vi "内置参数设置.vi"() -> ()   [LabVIEW 2016, in "斯坦道CODMn新电路板.lvlib"]
uses:
  <vilib>/Utility/miscctls.llb/LVPointTypeDef.ctl
panel:
  in  "传感器阈值:":u16
  in  "加速模式(速度):":u16
  in  "滴定延时时间:\n(单位:毫秒)":u16
  in  "斜率阈值:":dbl
  in  "阀配置:":u8(ring) items=["三通阀", "排阀"]
  in  "AB跨度告警值:":u16
  in  "B值告警上限值:":u16
  in  "B值范围:":u16
  in  "A值告警上限值:":u16
  in  "A值范围:":u16
  in  "是否存在液位检测板:":u16(ring) items=["否", "是"]
  in  "检出限(mg/L):":dbl
  in  "测量精度(mg/L):":dbl
  in  "ILimitDown":dbl
  in  "ILimitUp:":dbl
  in  "K d:":dbl
  in  "K i:":dbl
  in  "K p:":dbl
  in  "加热超时时间:(单位:秒)":dbl
  in  "告警温度:":dbl
  in  "加热温度:  校准参数":dbl
  in  "运行速度:  (修改需要重启)":u16
  in  "偏心轮: 校准参数":dbl
  in  "注射泵加热超时时间(s):":u16
  in  "注射泵保温温度H:":u8
  in  "注射泵\n保温温度L:":u8
  in  "废液通道:":u8
  in  "纯水通道:":u8
  in  "滴定速度:":u16
  in  "出样速度:":u16
  in  "进样速度:":u16
  in  "阀数量:":u8(ring) items=["9通"=9, "12通"=12]
  in  "注射泵型号":u8(ring) items=["TECAN", "润泽", "旋转阀"]
  in  "阈值(高→低)(mg/L):":dbl
  in  "阈值(低→高)(mg/L):":dbl
  in  "检测下限(mg/L):":dbl
  in  "检测上限(mg/L):":dbl
  in  "关闭":bool
  in  "保存":bool
  in  "读取":bool
  # "仪器内部参数设置"
  # "~"
  # "~"
  # "~"
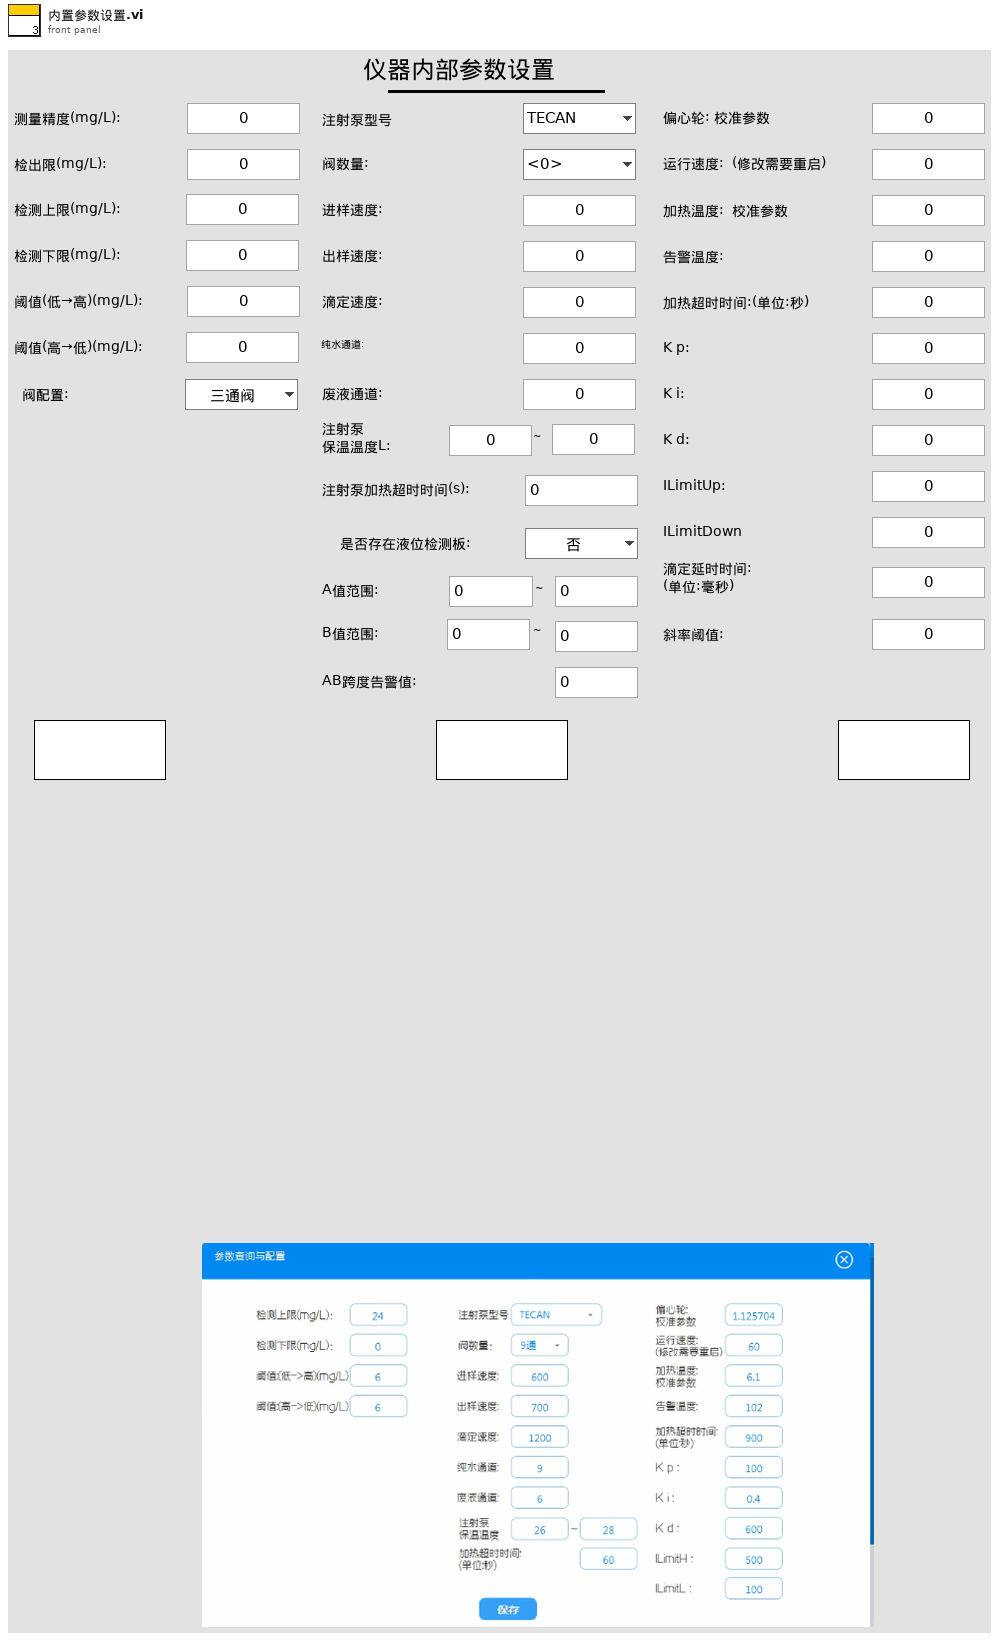
[diagram p1: front panel]
types:
  T1 = typedef "LVPointTypeDef.ctl" = cluster{"Horizontal":i16, "Vertical":i16}
  T2 = cluster{"偏心轮校准参数":dbl, "运行速度(修改需要重启)":u16, "加热温度(校准参数) ":dbl, "告警温度":dbl, "加热超时时间:(单位/秒)":dbl, "K p":dbl, "K i":dbl, "K d":dbl, "ILimitUp":dbl, "ILimitDown":dbl}
  T3 = cluster{"泵类型":u8, "阀数量":u8, "纯水通道":u8, "废液通道":u8, "进样速度":u16, "出样速度":u16, "滴定速度":u16, "注射泵保温温度L":u8, "注射泵保温温度H":u8, "注射泵加热超时时间":u16, "是否存在液位检测板":u16, "A值告警下限值":u16, "A值告警上限值":u16, "B值告警下限值":u16, "B值告警上限值":u16, "AB跨度告警值":u16, "阀配置:":u8, "滴定等待时间":u16, "滴定吸光度斜率":dbl, "传感器阈值":u16, "加速模式(速度):":u16}
  T4 = cluster{"检出限":dbl, "测量精度":dbl, "上限":dbl, "下限":dbl, "阈值（低->高）":dbl, "阈值（高->低）":dbl}
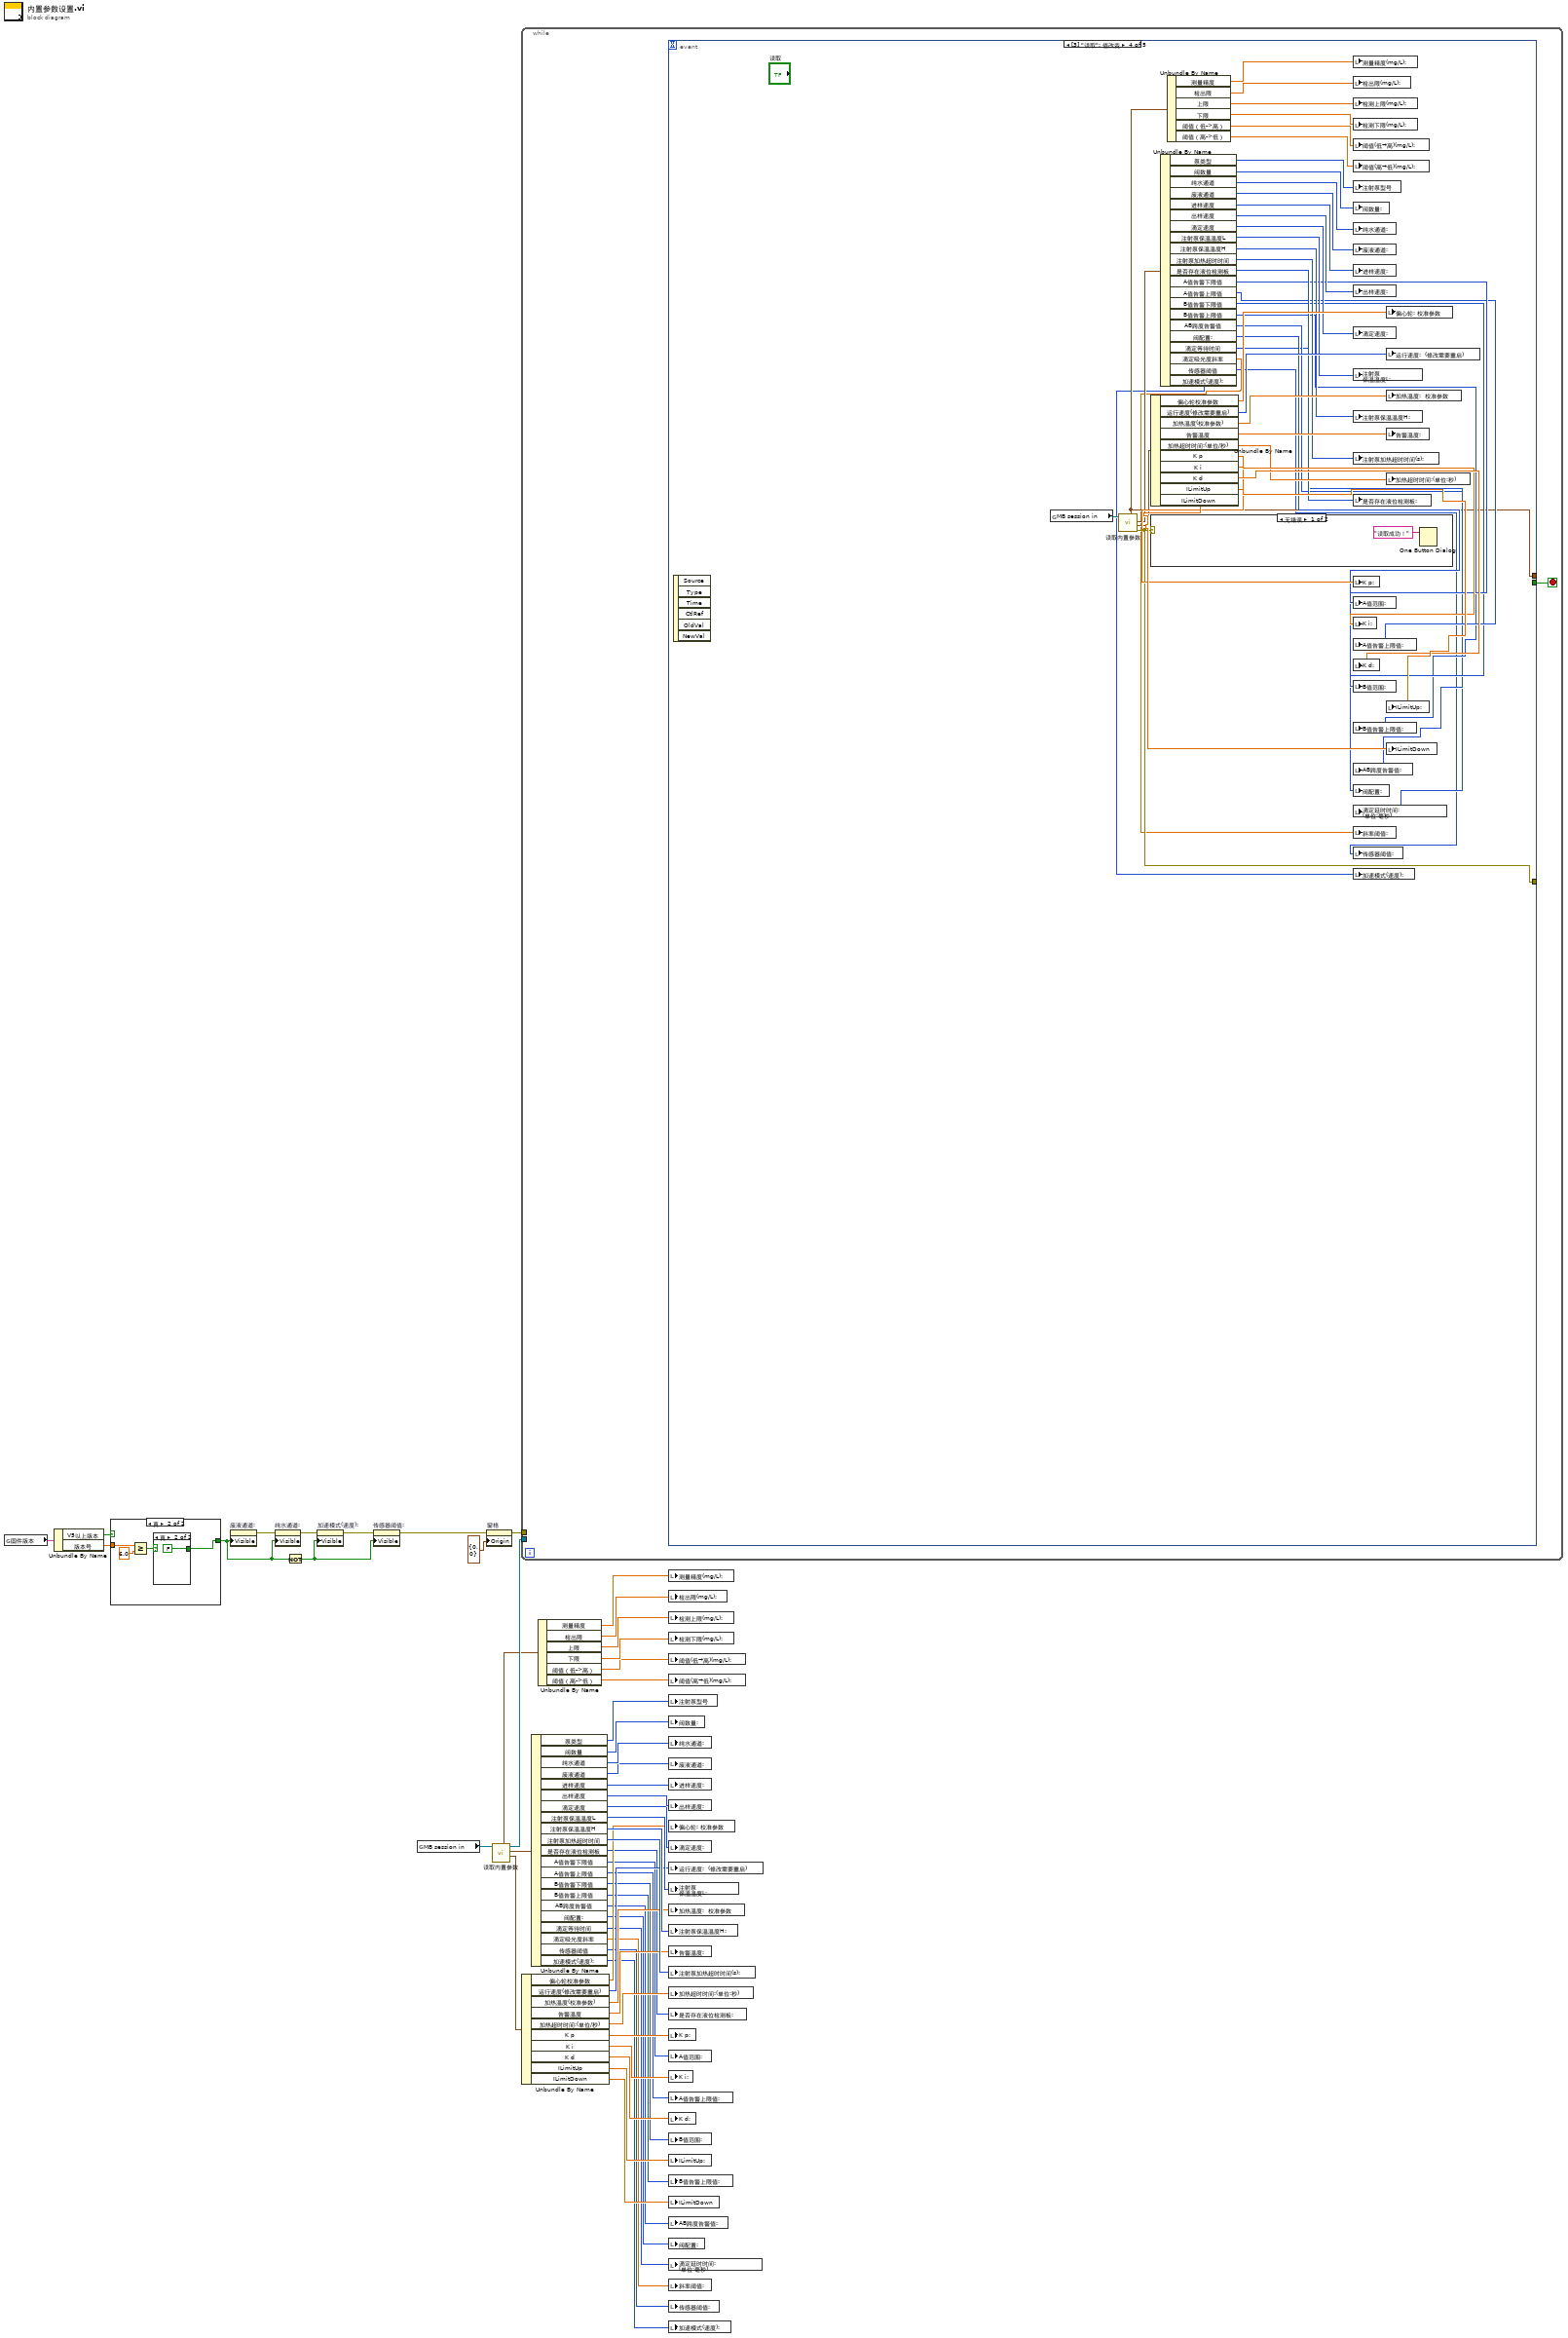
[diagram p0: block diagram]
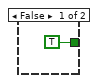
[diagram p2: hidden frame]
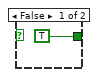
[diagram p3: hidden frame]
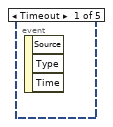
[diagram p4: hidden frame]
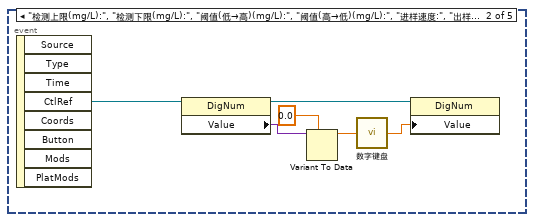
[diagram p5: hidden frame]
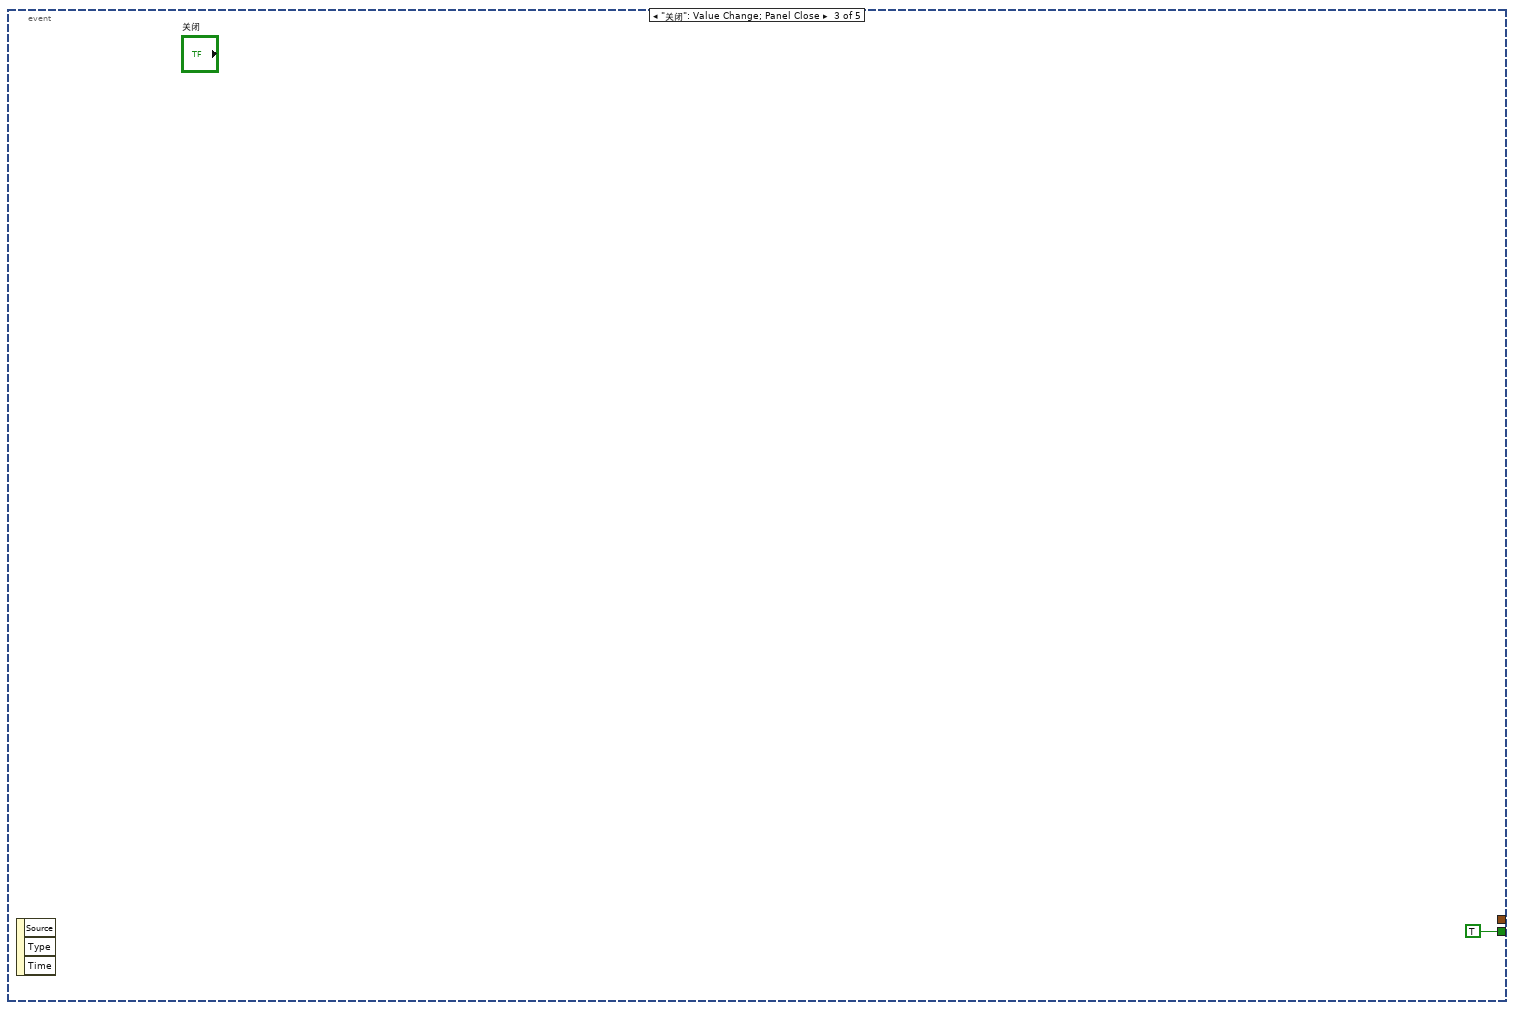
[diagram p6: hidden frame]
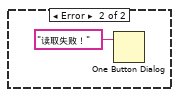
[diagram p7: hidden frame]
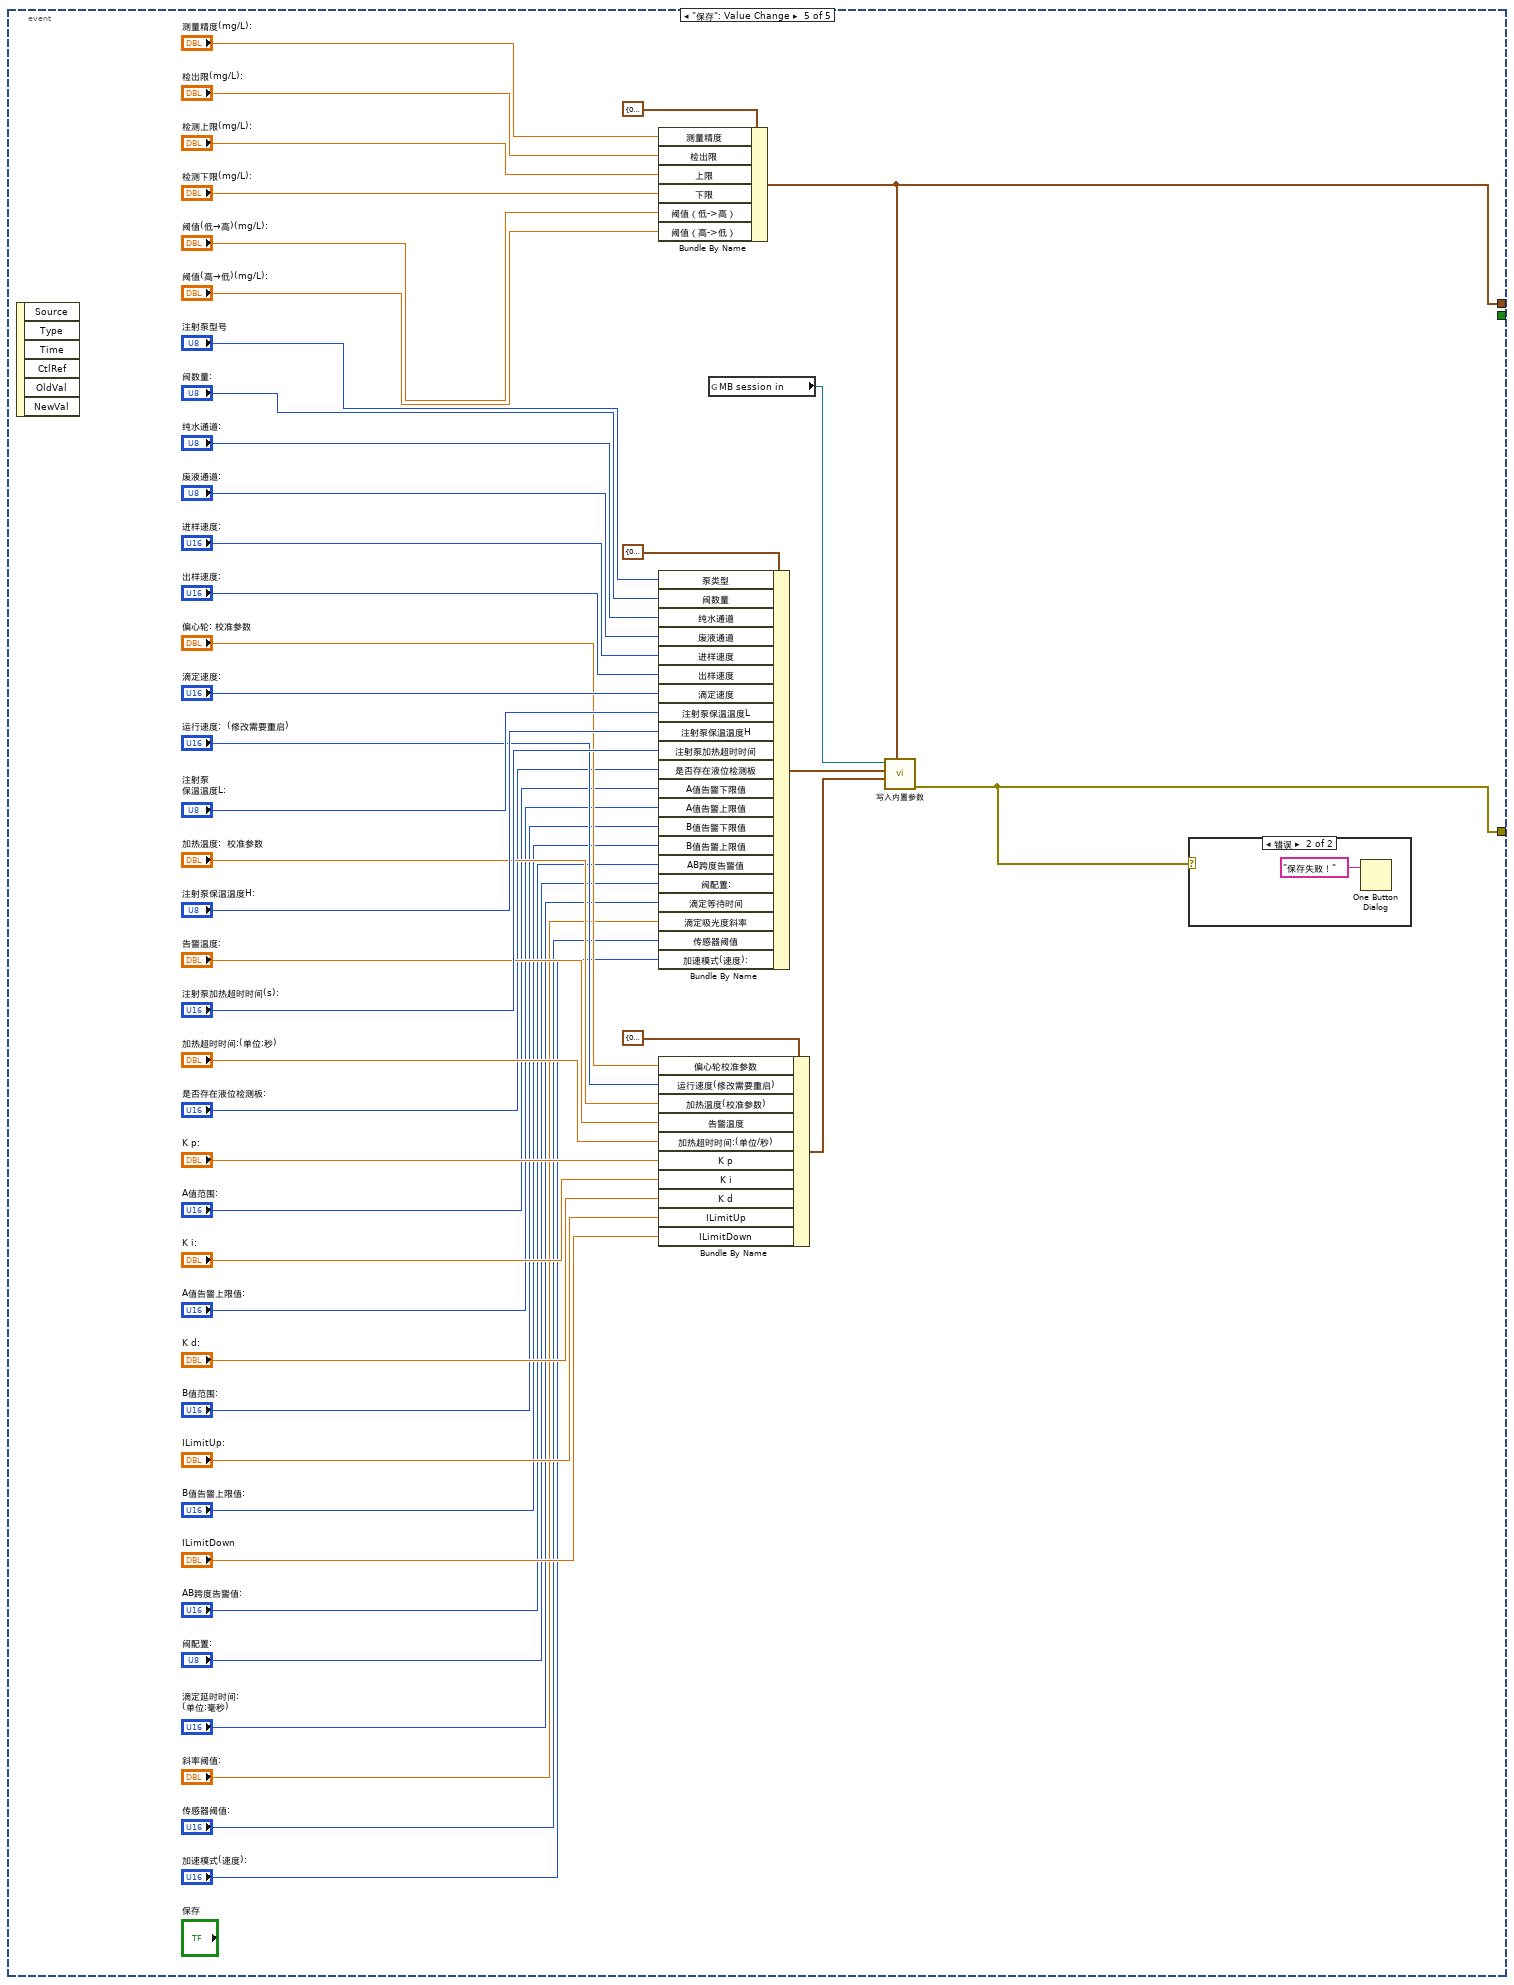
[diagram p8: hidden frame]
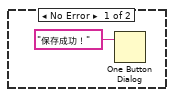
[diagram p9: hidden frame]
diagram:
  n1 = global read "VARCODMn全局变量.vi" "固件版本"() -> (w11:cluster{"V5以上版本":bool, "版本号":dbl})
  n2 = Unbundle By Name(w11) -> ("V5以上版本"=w10:bool, "版本号"=w9:dbl)
  n3 = case shown="真" w10 {
    tunnel: w9 -> [_ w57]
    tunnel: [TRUE w55] -> w6
    frame False {
    }
    frame True {
      n4 = Greater Or Equal?(x=w57, y=6.0) -> (x >= y?=w56:bool)
      n5 = case shown="真" w56 {
        tunnel: [TRUE FALSE] -> w55
        frame False {
        }
        frame True {
        }
      }
    }
  }
  n6 = property on="废液通道:" class="DigNum (严格)"("Visible"=w6) -> (error out=w8:errorcluster)  [unwired: 2 in, 1 out]
  n7 = property on="纯水通道:" class="DigNum (严格)"(error in=w8, "Visible"=w6) -> (error out=w7:errorcluster)  [unwired: 1 in, 1 out]
  n8 = Not(x=w6) -> (.not. x?=w4:bool)
  n9 = property on="加速模式(速度):" class="DigNum (严格)"(error in=w7, "Visible"=w4) -> (error out=w5:errorcluster)  [unwired: 1 in, 1 out]
  n10 = property on="传感器阈值:" class="DigNum (严格)"(error in=w5, "Visible"=w4) -> (error out=w3:errorcluster)  [unwired: 1 in, 1 out]
  n11 = global read "VARCODMn全局变量.vi" "MB session in"() -> (w51:refnum<class "MB_Master.lvclass">)
  n12 = property on="窗格" class="Pane"(error in=w3, "Origin"=T1 {"Horizontal"=0, "Vertical"=0} ("原点")) -> (error out=w52:errorcluster)  [unwired: 1 in, 1 out]
  n13 = call "读取内置参数.vi"("MB session in"=w51) -> ("float"=w48:T2, "外设配置"=w49:T3, "MB session out"=w50:refnum<class "MB_Master.lvclass">, "量程参数读取"=w14:T4)  [unwired: 6 in, 1 out]
  n14 = while {
    tunnel: w52 -> [_]
    tunnel: w50 -> [_]
    stop <- w61 stop-if-true
    n15 = event shown="[3] \"读取\": 值改变" {
      selector: _ -> [_ _ _ _ _]
      dyn-events: _ -> [_ _ _ _ _]
      timeout: _ -> [_ _ _ _ _]
      tunnel: [_ _ TRUE _ _] -> w61
      tunnel: [_ _ _ w81 w128] -> _
      tunnel: [_ _ _ w73 w119] -> _
      event Timeout {
        n16 = event-data() -> ()  [unwired: 1 in, 3 out]
      }
      event "检测上限(mg/L):", "检测下限(mg/L):", "阈值(低→高)(mg/L):", "阈值(高→低)(mg/L):", "进样速度:", "出样速度:", "滴定速度:", "纯水通道:", "废液通道:", "注射泵\n保温温度L:", "注射泵保温温度H:", "注射泵加热超时时间(s):", "偏心轮: 校准参数", "运行速度:  (修改需要重启)", "告警温度:", "加热温度:  校准参数", "K p:", "K i:", "K d:", "ILimitUp:", "ILimitDown", "测量精度(mg/L):", "检出限(mg/L):", "A值范围:", "A值告警上限值:", "B值范围:", "B值告警上限值:", "AB跨度告警值:", "斜率阈值:", "滴定延时时间:\n(单位:毫秒)", "加速模式(速度):", "传感器阈值:": Mouse Down {
        n17 = event-data() -> ("CtlRef"=w67:refnum<vi>)  [unwired: 1 in, 7 out]
        n18 = property class="DigNum"(reference=w67) -> (reference out=w66:refnum<vi>, "Value"=w64:variant)  [unwired: 1 in, 1 out]
        n19 = Variant To Data(type=0.0 ("OldNumber"), Variant=w64) -> (data=w62:dbl)  [unwired: 1 in, 1 out]
        n20 = call "数字键盘.vi"("OldNumber"=w62) -> ("NewNumber"=w65:dbl)
        n21 = property class="DigNum"(reference=w66, "Value"=w65) -> ()  [unwired: 1 in, 2 out]
      }
      event "关闭": Value Change; Panel Close {
        n22 = event-data() -> ()  [unwired: 1 in, 3 out]
      }
      event "读取": Value Change {
        n23 = event-data() -> ()  [unwired: 1 in, 6 out]
        n24 = global read "VARCODMn全局变量.vi" "MB session in"() -> (w82:refnum<class "MB_Master.lvclass">)
        n25 = call "读取内置参数.vi"("MB session in"=w82) -> ("error out"=w81:errorcluster, "float"=w84:T2, "外设配置"=w83:T3, "量程参数读取"=w73:T4)  [unwired: 6 in, 1 out]
        n26 = Unbundle By Name(w84) -> ("偏心轮校准参数"=w101:dbl, "运行速度(修改需要重启)"=w102:u16, "加热温度(校准参数)"=w103:dbl, "告警温度"=w104:dbl, "加热超时时间:(单位/秒)"=w105:dbl, "K p"=w106:dbl, "K i"=w107:dbl, "K d"=w108:dbl, "ILimitUp"=w109:dbl, "ILimitDown"=w110:dbl)
        n27 = case shown="无错误" w81 {
          frame No Error {
            n28 = One Button Dialog(message="读取成功！" ("消息")) -> ()  [unwired: 1 in, 1 out]
          }
          frame Error {
            n29 = One Button Dialog(message="读取失败！" ("消息")) -> ()  [unwired: 1 in, 1 out]
          }
        }
        n30 = Unbundle By Name(w83) -> ("泵类型"=w91:u8, "阀数量"=w92:u8, "纯水通道"=w93:u8, "废液通道"=w94:u8, "进样速度"=w95:u16, "出样速度"=w96:u16, "滴定速度"=w97:u16, "注射泵保温温度L"=w98:u8, "注射泵保温温度H"=w99:u8, "注射泵加热超时时间"=w100:u16, "是否存在液位检测板"=w80:u16, "A值告警下限值"=w79:u16, "A值告警上限值"=w78:u16, "B值告警下限值"=w77:u16, "B值告警上限值"=w76:u16, "AB跨度告警值"=w75:u16, "阀配置:"=w74:u8, "滴定等待时间"=w72:u16, "滴定吸光度斜率"=w71:dbl, "传感器阈值"=w70:u16, "加速模式(速度):"=w69:u16)
        n31 = Unbundle By Name(w73) -> ("测量精度"=w85:dbl, "检出限"=w86:dbl, "上限"=w87:dbl, "下限"=w88:dbl, "阈值（低->高）"=w89:dbl, "阈值（高->低）"=w90:dbl)
        n32 = local write "测量精度(mg/L):"(w85) -> ()
        n33 = local write "检出限(mg/L):"(w86) -> ()
        n34 = local write "检测上限(mg/L):"(w87) -> ()
        n35 = local write "检测下限(mg/L):"(w88) -> ()
        n36 = local write "阈值(低→高)(mg/L):"(w89) -> ()
        n37 = local write "阈值(高→低)(mg/L):"(w90) -> ()
        n38 = local write "注射泵型号"(w91) -> ()
        n39 = local write "阀数量:"(w92) -> ()
        n40 = local write "纯水通道:"(w93) -> ()
        n41 = local write "废液通道:"(w94) -> ()
        n42 = local write "进样速度:"(w95) -> ()
        n43 = local write "出样速度:"(w96) -> ()
        n44 = local write "滴定速度:"(w97) -> ()
        n45 = local write "注射泵\n保温温度L:"(w98) -> ()
        n46 = local write "注射泵保温温度H:"(w99) -> ()
        n47 = local write "注射泵加热超时时间(s):"(w100) -> ()
        n48 = local write "是否存在液位检测板:"(w80) -> ()
        n49 = local write "K p:"(w106) -> ()
        n50 = local write "A值范围:"(w79) -> ()
        n51 = local write "K i:"(w107) -> ()
        n52 = local write "A值告警上限值:"(w78) -> ()
        n53 = local write "K d:"(w108) -> ()
        n54 = local write "B值范围:"(w77) -> ()
        n55 = local write "B值告警上限值:"(w76) -> ()
        n56 = local write "AB跨度告警值:"(w75) -> ()
        n57 = local write "阀配置:"(w74) -> ()
        n58 = local write "滴定延时时间:\n(单位:毫秒)"(w72) -> ()
        n59 = local write "斜率阈值:"(w71) -> ()
        n60 = local write "传感器阈值:"(w70) -> ()
        n61 = local write "加速模式(速度):"(w69) -> ()
        n62 = local write "偏心轮: 校准参数"(w101) -> ()
        n63 = local write "运行速度:  (修改需要重启)"(w102) -> ()
        n64 = local write "加热温度:  校准参数"(w103) -> ()
        n65 = local write "告警温度:"(w104) -> ()
        n66 = local write "加热超时时间:(单位:秒)"(w105) -> ()
        n67 = local write "ILimitUp:"(w109) -> ()
        n68 = local write "ILimitDown"(w110) -> ()
      }
      event "保存": Value Change {
        n69 = event-data() -> ()  [unwired: 1 in, 6 out]
        n70 = Bundle By Name(cluster=T4 {"检出限"=0.0, "测量精度"=0.0, "上限"=0.0, "下限"=0.0, "阈值（低->高）"=0.0, "阈值（高->低）"=0.0} ("量程参数读取"), "测量精度"="测量精度(mg/L):", "检出限"="检出限(mg/L):", "上限"="检测上限(mg/L):", "下限"="检测下限(mg/L):", "阈值（低->高）"="阈值(低→高)(mg/L):", "阈值（高->低）"="阈值(高→低)(mg/L):") -> (w119:T4)
        n71 = Bundle By Name(cluster=T3 {"泵类型"=0, "阀数量"=0, "纯水通道"=0, "废液通道"=0, "进样速度"=0, "出样速度"=0, "滴定速度"=0, "注射泵保温温度L"=0, "注射泵保温温度H"=0, "注射泵加热超时时间"=0, "是否存在液位检测板"=0, "A值告警下限值"=0, "A值告警上限值"=0, "B值告警下限值"=0, "B值告警上限值"=0, "AB跨度告警值"=0, "阀配置:"=0, "滴定等待时间"=0, "滴定吸光度斜率"=0.0, "传感器阈值"=0, "加速模式(速度):"=0} ("外设配置"), "泵类型"="注射泵型号", "阀数量"="阀数量:", "纯水通道"="纯水通道:", "废液通道"="废液通道:", "进样速度"="进样速度:", "出样速度"="出样速度:", "滴定速度"="滴定速度:", "注射泵保温温度L"="注射泵\n保温温度L:", "注射泵保温温度H"="注射泵保温温度H:", "注射泵加热超时时间"="注射泵加热超时时间(s):", "是否存在液位检测板"="是否存在液位检测板:", "A值告警下限值"="A值范围:", "A值告警上限值"="A值告警上限值:", "B值告警下限值"="B值范围:", "B值告警上限值"="B值告警上限值:", "AB跨度告警值"="AB跨度告警值:", "阀配置:"="阀配置:", "滴定等待时间"="滴定延时时间:\n(单位:毫秒)", "滴定吸光度斜率"="斜率阈值:", "传感器阈值"="传感器阈值:", "加速模式(速度):"="加速模式(速度):") -> (w117:T3)
        n72 = Bundle By Name(cluster=T2 {"偏心轮校准参数"=0.0, "运行速度(修改需要重启)"=0, "加热温度(校准参数) "=0.0, "告警温度"=0.0, "加热超时时间:(单位/秒)"=0.0, "K p"=0.0, "K i"=0.0, "K d"=0.0, "ILimitUp"=0.0, "ILimitDown"=0.0} ("float"), "偏心轮校准参数"="偏心轮: 校准参数", "运行速度(修改需要重启)"="运行速度:  (修改需要重启)", "加热温度(校准参数)"="加热温度:  校准参数", "告警温度"="告警温度:", "加热超时时间:(单位/秒)"="加热超时时间:(单位:秒)", "K p"="K p:", "K i"="K i:", "K d"="K d:", "ILimitUp"="ILimitUp:", "ILimitDown"="ILimitDown") -> (w129:T2)
        n73 = global read "VARCODMn全局变量.vi" "MB session in"() -> (w157:refnum<class "MB_Master.lvclass">)
        n74 = call "写入内置参数.vi"("量程参数读取"=w119, "float"=w129, "外设配置"=w117, "MB session in"=w157) -> ("error out"=w128:errorcluster)  [unwired: 6 in, 1 out]
        n75 = case shown="错误" w128 {
          frame No Error {
            n76 = One Button Dialog(message="保存成功！" ("消息")) -> ()  [unwired: 1 in, 1 out]
          }
          frame Error {
            n77 = One Button Dialog(message="保存失败！" ("消息")) -> ()  [unwired: 1 in, 1 out]
          }
        }
      }
    }
  }
  n78 = Unbundle By Name(w48) -> ("偏心轮校准参数"=w31:dbl, "运行速度(修改需要重启)"=w30:u16, "加热温度(校准参数)"=w29:dbl, "告警温度"=w28:dbl, "加热超时时间:(单位/秒)"=w27:dbl, "K p"=w26:dbl, "K i"=w25:dbl, "K d"=w24:dbl, "ILimitUp"=w23:dbl, "ILimitDown"=w22:dbl)
  n79 = Unbundle By Name(w49) -> ("泵类型"=w41:u8, "阀数量"=w40:u8, "纯水通道"=w39:u8, "废液通道"=w38:u8, "进样速度"=w37:u16, "出样速度"=w36:u16, "滴定速度"=w35:u16, "注射泵保温温度L"=w34:u8, "注射泵保温温度H"=w33:u8, "注射泵加热超时时间"=w32:u16, "是否存在液位检测板"=w21:u16, "A值告警下限值"=w20:u16, "A值告警上限值"=w19:u16, "B值告警下限值"=w18:u16, "B值告警上限值"=w17:u16, "AB跨度告警值"=w16:u16, "阀配置:"=w15:u8, "滴定等待时间"=w12:u16, "滴定吸光度斜率"=w13:dbl, "传感器阈值"=w2:u16, "加速模式(速度):"=w1:u16)
  n80 = Unbundle By Name(w14) -> ("测量精度"=w47:dbl, "检出限"=w46:dbl, "上限"=w45:dbl, "下限"=w44:dbl, "阈值（低->高）"=w43:dbl, "阈值（高->低）"=w42:dbl)
  n81 = local write "测量精度(mg/L):"(w47) -> ()
  n82 = local write "检出限(mg/L):"(w46) -> ()
  n83 = local write "检测上限(mg/L):"(w45) -> ()
  n84 = local write "检测下限(mg/L):"(w44) -> ()
  n85 = local write "阈值(低→高)(mg/L):"(w43) -> ()
  n86 = local write "阈值(高→低)(mg/L):"(w42) -> ()
  n87 = local write "注射泵型号"(w41) -> ()
  n88 = local write "阀数量:"(w40) -> ()
  n89 = local write "纯水通道:"(w39) -> ()
  n90 = local write "废液通道:"(w38) -> ()
  n91 = local write "进样速度:"(w37) -> ()
  n92 = local write "出样速度:"(w36) -> ()
  n93 = local write "偏心轮: 校准参数"(w31) -> ()
  n94 = local write "滴定速度:"(w35) -> ()
  n95 = local write "运行速度:  (修改需要重启)"(w30) -> ()
  n96 = local write "注射泵\n保温温度L:"(w34) -> ()
  n97 = local write "加热温度:  校准参数"(w29) -> ()
  n98 = local write "注射泵保温温度H:"(w33) -> ()
  n99 = local write "告警温度:"(w28) -> ()
  n100 = local write "注射泵加热超时时间(s):"(w32) -> ()
  n101 = local write "加热超时时间:(单位:秒)"(w27) -> ()
  n102 = local write "是否存在液位检测板:"(w21) -> ()
  n103 = local write "K p:"(w26) -> ()
  n104 = local write "A值范围:"(w20) -> ()
  n105 = local write "K i:"(w25) -> ()
  n106 = local write "A值告警上限值:"(w19) -> ()
  n107 = local write "K d:"(w24) -> ()
  n108 = local write "B值范围:"(w18) -> ()
  n109 = local write "ILimitUp:"(w23) -> ()
  n110 = local write "B值告警上限值:"(w17) -> ()
  n111 = local write "ILimitDown"(w22) -> ()
  n112 = local write "AB跨度告警值:"(w16) -> ()
  n113 = local write "阀配置:"(w15) -> ()
  n114 = local write "滴定延时时间:\n(单位:毫秒)"(w12) -> ()
  n115 = local write "斜率阈值:"(w13) -> ()
  n116 = local write "传感器阈值:"(w2) -> ()
  n117 = local write "加速模式(速度):"(w1) -> ()
